vi "SMO.CastArrayDependenciesToCluster.vi"(7 "{Dependencies Type}":variant, 8 "error in (no error)":errorcluster, 11 "[Dependencies]":refnum<class "SMO.lvclass">[](array[class])) -> (0 "error out":errorcluster, 3 "Dependencies Cluster":variant)   [LabVIEW 2013, in "SMO.lvclass"]
uses:
  SMO.lvclass
  <vilib>/Utility/VariantDataType/VariantType.lvlib
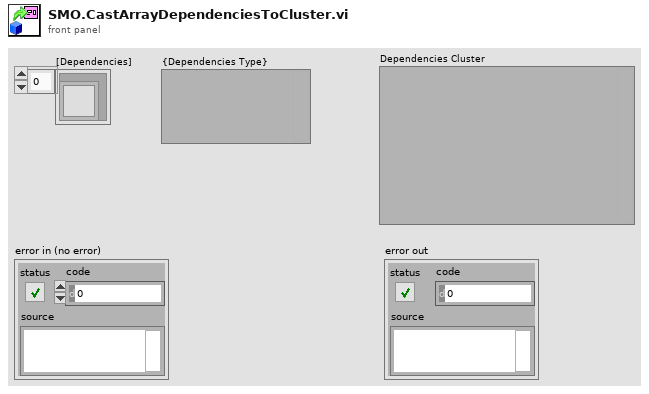
[diagram p1: front panel]
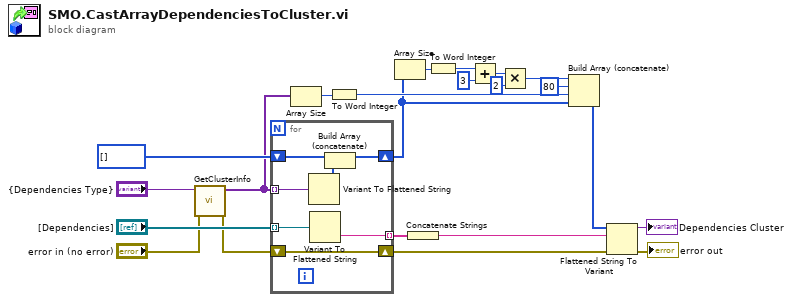
[diagram p0: block diagram]
diagram:
  n1 = call <vilib>:"GetClusterInfo.vi"("error in (no error)"="error in (no error)", "Variant"="{Dependencies Type}") -> ("error out"=w17:errorcluster, "Cluster Elements"=w15:variant[])  [unwired: 8 in]
  n2 = for {
    tunnel: "[Dependencies]" -> [w29] mode=indexing
    shift-right: [w28] -> w20
    shift-left: w17 -> [w28]
    tunnel: w15 -> [w27] mode=indexing
    shift-right: [w25] -> w3
    shift-left: i16[] [] -> [w26]
    tunnel: [w24] -> w11 mode=indexing
    n3 = Variant To Flattened String(Variant=w27) -> (1:w23:i16[])  [unwired: 1 out]
    n4 = Variant To Flattened String(Variant=w29) -> (data string=w24:string)  [unwired: 1 out]
    n5 = Build Array (concatenate)(w26, w23) -> (w25:i16[])
  }
  n6 = Array Size(array=w15) -> (size(s)=w14:i32)
  n7 = To Word Integer(number=w14) -> (16bit integer=w13:i16)
  n8 = Array Size(array=w3) -> (size(s)=w5:i32)
  n9 = Concatenate Strings(w11) -> (w10:string)
  n10 = To Word Integer(number=w5) -> (16bit integer=w9:i16)
  n11 = Add(x=w9, y=i16 3) -> (x+y=w7:i16)
  n12 = Multiply(x=w7, y=i16 2) -> (x*y=w4:i16)
  n13 = Build Array (concatenate)(w4, i16 80 ("16bit integer"), w13, w3) -> (w2:i16[])
  n14 = Flattened String To Variant(4:w20, 6:w10, 7:w2) -> (0:→"error out":errorcluster, 3:→"Dependencies Cluster":variant)
